vi "PH_Sequencer.PC CheckHeads.vi"(0 "i ref in":refnum<vi>, 5 "error in (no error)":errorcluster) -> (14 "i ref out":refnum<vi>, 19 "error out":errorcluster)   [LabVIEW 2014, in "PH_Sequencer.lvlib"]
doc: "This VI checks wether the heads are ready for shot."
uses:
  PH_Sequencer.lvlib
  PH_Basics/PH_PP_Common/PH_PP_Common.PUs.ctl
  PH_Basics/PH_PowerUnit_BaseClass/PH_PowerUnit_BaseClass.SM States.ctl
  PH_Basics/PH_Common/PH_Common.lvlib
  PH_BeamlineInformation/PH_BeamlineInformation.lvlib
  PH_Basics/PH_PP_Common/PH_PP_Common.lvlib
  PH_Basics/PH_PowerUnit_BaseClass/PH_PowerUnit_BaseClass.lvlib
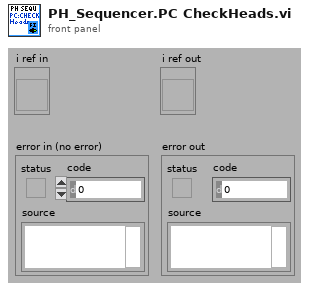
[diagram p1: front panel]
types:
  T1 = typedef "PH_PP_Common.lvlib/PH_PP_Common.PUs.ctl" = enum16{"no Info", "PA-19mm-1", "PA-19mm-2", "PA-45mm-PILC", "PA-45mm-MAIN", "MA-PU-1", "MA-PU-2", "MA-PU-3", "MA-PU-4", "MA-PU-5", "MA-PU-6", "MA-FR", "MA-PILC", "PA-45mm-DP"}
  T2 = typedef "PH_BeamlineInformation.lvlib/PH_BeamlineInformation.i attribute.ctl" = cluster{"BL GUI Elements of Services":cluster{"Service Name":string, "GUI Elements":refnum<vi>[], "Status":i32}[], "Powermeters":T3, "Efficiency":T4, "Heads":T5[]}
  T3 = typedef "PH_BeamlineInformation.lvlib/PH_BeamlineInformation.Powermeter.ctl" = cluster{"ns FE":cluster{"GUI Ref":refnum<vi>, "Value":dbl}, "fs FE":cluster{"GUI Ref":refnum<vi>, "Value":dbl}, "PA":cluster{"GUI Ref":refnum<vi>, "Value":dbl}, "MA":cluster{"GUI Ref":refnum<vi>, "Value":dbl}, "Z6 green":cluster{"GUI Ref":refnum<vi>, "Value":dbl}, "Z6 IR":cluster{"GUI Ref":refnum<vi>, "Value":dbl}, "Z6 COS":cluster{"GUI Ref":refnum<vi>, "Value":dbl}}
  T4 = typedef "PH_BeamlineInformation.lvlib/PH_BeamlineInformation.Efficiency.ctl" = cluster{"PA Gain":cluster{"GUI Ref":refnum<vi>, "Value":dbl}, "MA Gain":cluster{"GUI Ref":refnum<vi>, "Value":dbl}, "Z6 green Conversion":cluster{"GUI Ref":refnum<vi>, "Value":dbl}, "Z6 Comp Losses":cluster{"GUI Ref":refnum<vi>, "Value":dbl}}
  T5 = typedef "PH_BeamlineInformation.lvlib/PH_BeamlineInformation.Head.ctl" = cluster{"PowerUnit":T1, "in use":cluster{"Value":bool, "GUI Ref":refnum<vi>, "linked":bool}, "voltage":cluster{"Value":dbl, "GUI Ref":refnum<vi>, "linked":bool}}
  T6 = typedef "PH_Sequencer.lvlib/PH_Sequencer.i attribute.ctl" = cluster{"GUI Refs":cluster{"Main Off":refnum<vi>, "Fire":refnum<vi>, "Status":refnum<vi>, "Ready":refnum<vi>, "Waiting Time":refnum<vi>, "Timeout":refnum<vi>, "PPMA Ready":refnum<vi>, "Sequencer SM State":refnum<vi>, "PPPA Ready":refnum<vi>, "Calorimeter":refnum<vi>, "Beamline Ready":refnum<vi>, "Clear Beamline":refnum<vi>, "Linkage PPMA Rods":refnum<vi>, "Linkage Current PA":refnum<vi>, "Linkage Current MA":refnum<vi>, "Timing Ready":refnum<vi>, "State Timing":refnum<vi>, "Force Timing":refnum<vi>, "PSDB Shot Comment":refnum<vi>, "State PA Backreflection":refnum<vi>, "Beamline Z6 Ready":refnum<vi>, "Clear Z6 Beamline":refnum<vi>, "Sequence length":refnum<vi>, "Timing Mode":refnum<vi>, "Slow Trigger Settings":refnum<vi>, "Experiment Description":refnum<vi>, "State PSDB":refnum<vi>, "PSDB Ready":refnum<vi>, "Set PSDB Settings":refnum<vi>, "Get PSDB Info":refnum<vi>, "Take Snapshot":refnum<vi>, "Shottype":refnum<vi>, "Experiment":refnum<vi>, "Phase Frontends":refnum<vi>, "PP 45mm PILC in use":refnum<vi>}, "Status Info":cluster{"Machine Status":T7, "WaitingTime":i32, "Timeout":bool}, "Readyness":cluster{"Ready to shot":bool, "PPMA Ready":bool, "PPPA Ready":bool, "BL Ready":bool, "Timing Ready":bool, "BL Z6 Ready":bool, "PSDBReady":bool}, "Instancenames":cluster{"PPMA Rods":string, "PP Current Meas":string, "PH Beamline Chief":string, "PA Backrefl Meas":string, "Z6 Beamline Chief":string}, "Data to read":bool, "Calorimeter":cluster{"Instancename":string, "On":bool, "linked":bool}, "Linkage":cluster{"PPMA Rods":bool, "PP Current Meas":bool, "PHELIX Beamline Chief":bool, "PA Backrefl Meas":bool, "Z6 Beamline Chief":bool}, "Timing":cluster{"Instance":string, "linked":bool, "Status":T7, "Timing Mode":T8, "Slow Trigger Settings":T9, "Info available":cluster{"ext SlowTrigger":bool, "T2":bool, "Mode":bool, "Delay Slow Trigger":bool, "Phase FEs":bool}, "FE Phase":T10}, "Service ID R2S":i32, "PSDB":cluster{"Controller Instance":string, "Controller Status":T7, "Controller linked":bool, "Settings acknowledged":bool, "Current Experiment ID":i16, "Current Shot Type":i16, "Current Comment":string, "Remember Settings":bool, "Write 2 early":bool}, "PSDB Data":cluster{"Main Off?":bool, "Sequence Length":dbl, "Sequence startet":timestamp}, "6P 4Q Positions":cluster{"Instancename":string, "linked":bool, "Position":T11}[], "PUs":T12[]}
  T7 = typedef "PH_StatusHandler.lvlib/PH_StatusHandler.Status.ctl" = i16
  T8 = typedef "PH_Timing.lvlib/PH_Timing.Timing Mode.ctl" = cluster{"T2":i16, "Modeselector":enum32{"10 Hz", "0.5 Hz", "Shot"}}
  T9 = typedef "PH_Timing.lvlib/PH_Timing.Slow Trigger Settings.ctl" = cluster{"Delay":dbl, "externally triggered?":bool}
  T10 = typedef "PH_Timing.lvlib/PH_Timing.Phase FEs.ctl" = cluster{"Phase":dbl}
  T11 = typedef "PH_4_Pos_Selector.lvlib/PH_4_Pos_Selector.Position Selector.ctl" = u16
  T12 = typedef "PH_Sequencer.lvlib/PH_Sequencer.Head.ctl" = cluster{"PowerUnit":T1, "GUI Ref":refnum<vi>, "Information":T13, "linked?":bool, "GUI Ref Current Voltage":refnum<vi>}
  T13 = typedef "PH_Sequencer.lvlib/PH_Sequencer.PU Information.ctl" = cluster{"State":T7, "Waiting Time [s]":dbl, "PU State SM":T14, "PU Timeout SM":T14}
  T14 = typedef "PH_PowerUnit_BaseClass.lvlib/PH_PowerUnit_BaseClass.SM States.ctl" = enum16{".", "Stand by", "Switch PU on", "Configure", "Set Default Voltage", "Set STANDBY", "Set READY", "Wait for Shot Cmd", "Open Dump Rods", "Open Ross Relais", "Close Ross Relais", "Switch PSU on", "Switch PSU off", "Charge", "Switch GD Channel on", "Close Dump Rods", "Rods-TO", "RR-TO", "PSU-TO", "Trigger-TO"}
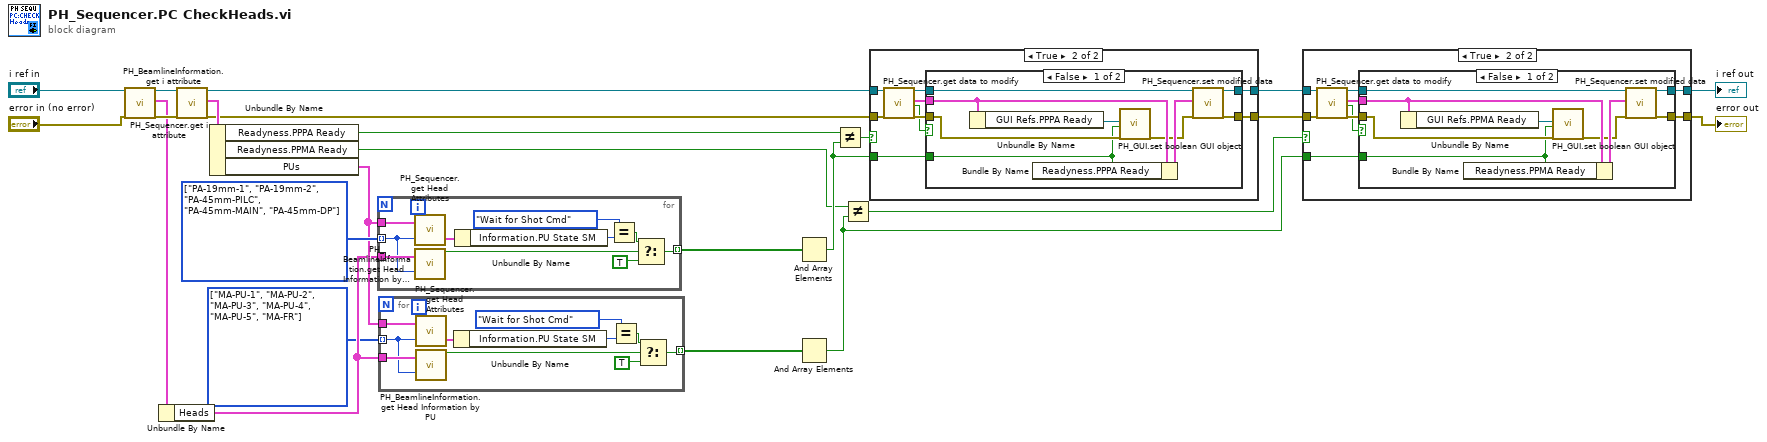
[diagram p0: block diagram]
diagram:
  w13 = T1[] [enum."PA-19mm-1", enum."PA-19mm-2", enum."PA-45mm-PILC", enum."PA-45mm-MAIN", enum."PA-45mm-DP"] items=["no Info", "PA-19mm-1", "PA-19mm-2", "PA-45mm-PILC", "PA-45mm-MAIN", "MA-PU-1", "MA-PU-2", "MA-PU-3", "MA-PU-4", "MA-PU-5", "MA-PU-6", "MA-FR", "MA-PILC", "PA-45mm-DP"]
  w1 = T1[] [enum."MA-PU-1", enum."MA-PU-2", enum."MA-PU-3", enum."MA-PU-4", enum."MA-PU-5", enum."MA-FR"] items=["no Info", "PA-19mm-1", "PA-19mm-2", "PA-45mm-PILC", "PA-45mm-MAIN", "MA-PU-1", "MA-PU-2", "MA-PU-3", "MA-PU-4", "MA-PU-5", "MA-PU-6", "MA-FR", "MA-PILC", "PA-45mm-DP"]
  n1 = call "PH_BeamlineInformation.get i attribute.vi"("i ref in"="i ref in", "error in (no error)"="error in (no error)") -> ("i ref out"=w20:refnum<vi>, "i attribute"=w19:T2, "error out"=w22:errorcluster)  [unwired: 15 in]
  n2 = Unbundle By Name(w19) -> ("Heads"=w10:T5[])
  n3 = call "PH_Sequencer.get i attribute.vi"("i ref in"=w20, "error in (no error)"=w22) -> ("i ref out"=w24:refnum<vi>, "i attribute"=w18:T6, "error out"=w14:errorcluster)  [unwired: 15 in]
  n4 = Unbundle By Name(w18) -> ("Readyness.PPPA Ready"=w16:bool, "Readyness.PPMA Ready"=w15:bool, "PUs"=w11:T12[])
  n5 = for {
    tunnel: w11 -> [w34]
    tunnel: w10 -> [w33]
    tunnel: w13 -> [w32] mode=indexing
    tunnel: [w27] -> w12 mode=indexing
    n6 = call "PH_Sequencer.get Head Attributes.vi"("PowerUnit"=w32, "Heads"=w34) -> ("Head"=w31:T12)  [unwired: 1 out]
    n7 = call "PH_BeamlineInformation.get Head Information by PU.vi"("Heads"=w33, "Power Unit"=w32) -> ("In Use?"=w30:bool)  [unwired: 12 in, 5 out]
    n8 = Unbundle By Name(w31) -> ("Information.PU State SM"=w29:T14)
    n9 = Equal?(x=PH_PowerUnit_BaseClass.SM_States."Wait for Shot Cmd", y=w29) -> (x = y?=w26:bool)
    n10 = Select(t=w26, s=w30, f=TRUE) -> (s? t:f=w27:bool)
  }
  n11 = for {
    tunnel: w11 -> [w44]
    tunnel: w10 -> [w43]
    tunnel: w1 -> [w42] mode=indexing
    tunnel: [w37] -> w9 mode=indexing
    n12 = call "PH_Sequencer.get Head Attributes.vi"("PowerUnit"=w42, "Heads"=w44) -> ("Head"=w41:T12)  [unwired: 1 out]
    n13 = call "PH_BeamlineInformation.get Head Information by PU.vi"("Heads"=w43, "Power Unit"=w42) -> ("In Use?"=w40:bool)  [unwired: 12 in, 5 out]
    n14 = Unbundle By Name(w41) -> ("Information.PU State SM"=w39:T14)
    n15 = Equal?(x=PH_PowerUnit_BaseClass.SM_States."Wait for Shot Cmd", y=w39) -> (x = y?=w36:bool)
    n16 = Select(t=w36, s=w40, f=TRUE) -> (s? t:f=w37:bool)
  }
  n17 = And Array Elements(Boolean array=w12) -> (logical AND=w17:bool)
  n18 = And Array Elements(Boolean array=w9) -> (logical AND=w2:bool)
  n19 = Not Equal?(x=w16, y=w17) -> (x != y?=w8:bool)
  n20 = Not Equal?(x=w15, y=w2) -> (x != y?=w3:bool)
  n21 = case shown="True" w8 {
    tunnel: [w45 w54] -> w5
    tunnel: [w46 w52] -> w7
    tunnel: w24 -> [w46 w49]
    tunnel: w14 -> [w45 w48]
    tunnel: w17 -> [_ w47]
    frame False {
    }
    frame True {
      n22 = call "PH_Sequencer.get data to modify.vi"("i ref in"=w49, "error in (no error)"=w48) -> ("i ref out"=w53:refnum<vi>, "i attribute"=w51:T6, "timed out"=w50:bool, "error out"=w55:errorcluster)  [unwired: 14 in]
      n23 = case shown="False" w50 {
        tunnel: w55 -> [w58 w65]
        tunnel: [w64 w65] -> w54
        tunnel: w53 -> [w63 w66]
        tunnel: [w62 w66] -> w52
        tunnel: w51 -> [w61 _]
        tunnel: w47 -> [w57 _]
        frame False {
          n24 = Unbundle By Name(w61) -> ("GUI Refs.PPPA Ready"=w59:refnum<vi>)
          n25 = Bundle By Name(cluster=w61, "Readyness.PPPA Ready"=w57) -> (w60:T6)
          n26 = call "PH_GUI.set boolean GUI object.vi"("Boolean Knob GUI Ref"=w59, "Value"=w57, "error in (no error)"=w58) -> ("error out"=w56:errorcluster)  [unwired: 16 in]
          n27 = call "PH_Sequencer.set modified data.vi"("i ref in"=w63, "i attribute"=w60, "error in (no error)"=w56) -> ("i ref out"=w62:refnum<vi>, "error out"=w64:errorcluster)  [unwired: 15 in]
        }
        frame True {
        }
      }
    }
  }
  n28 = case shown="True" w3 {
    tunnel: [w67 w76] -> w4
    tunnel: [w68 w74] -> w6
    tunnel: w7 -> [w68 w71]
    tunnel: w5 -> [w67 w70]
    tunnel: w2 -> [_ w69]
    frame False {
    }
    frame True {
      n29 = call "PH_Sequencer.get data to modify.vi"("i ref in"=w71, "error in (no error)"=w70) -> ("i ref out"=w75:refnum<vi>, "i attribute"=w73:T6, "timed out"=w72:bool, "error out"=w77:errorcluster)  [unwired: 14 in]
      n30 = case shown="False" w72 {
        tunnel: w77 -> [w80 w87]
        tunnel: [w86 w87] -> w76
        tunnel: w75 -> [w85 w88]
        tunnel: [w84 w88] -> w74
        tunnel: w73 -> [w83 _]
        tunnel: w69 -> [w79 _]
        frame False {
          n31 = Unbundle By Name(w83) -> ("GUI Refs.PPMA Ready"=w81:refnum<vi>)
          n32 = Bundle By Name(cluster=w83, "Readyness.PPMA Ready"=w79) -> (w82:T6)
          n33 = call "PH_GUI.set boolean GUI object.vi"("Boolean Knob GUI Ref"=w81, "Value"=w79, "error in (no error)"=w80) -> ("error out"=w78:errorcluster)  [unwired: 16 in]
          n34 = call "PH_Sequencer.set modified data.vi"("i ref in"=w85, "i attribute"=w82, "error in (no error)"=w78) -> ("i ref out"=w84:refnum<vi>, "error out"=w86:errorcluster)  [unwired: 15 in]
        }
        frame True {
        }
      }
    }
  }
  "i ref out" <- w6
  "error out" <- w4
